vi "Keithley6221Monitor.vi"() -> ()   [LabVIEW 2019]
uses:
  Utility/Monitor Communication/K6221/K6221_Cluster.ctl
  Global/Global Variables/Data_Display_global.vi
  Instrument_Setup.vi
  Utility/Monitor Communication/sub-vis/K6221_Open_Queue.vi
  Utility/Monitor Communication/sub-vis/K6221_Check_Queue.vi
  <vilib>/ErrorRing/Error Ring.xnode
  Equipment/Keithley 622x/Keithley 622x.lvlib
panel:
  out "Cluster":T1
  # "K 6221"
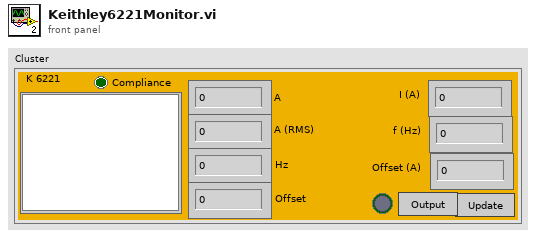
[diagram p1: front panel]
types:
  T1 = typedef "K6221_Cluster.ctl" = cluster{"Plot Window":dbl[][], "A":dbl, "A (RMS)":dbl, "Hz":dbl, "I (A)":dbl, "f (Hz)":dbl, "Update":bool, "Offset":dbl, "Offset (A)":dbl, "Compliance":bool, "Output":bool, "Output Status":bool}
  T2 = typedef "Keithley 622x.lvlib/KE622x -- Current Level.ctl" = dbl
  T3 = typedef "Keithley 622x.lvlib/KE622x -- On Off Control.ctl" = enum16{"Off", "On"}
  T4 = typedef "Keithley 622x.lvlib/KE6221 -- Wave Sine Wave Params.ctl" = cluster{"Frequency (Hz)":T5, "Amplitude (A)":T6, "Offset (A)":T2, "Ranging Mode":T7, "Fixed Range":T8, "Playback Mode":T9, "Time (s)":T10, "Num Cycles":T11, "Phase\nMarker?":bool, "Phase Marker (deg)":T12, "Trig Link Line":T13}
  T5 = typedef "Keithley 622x.lvlib/KE6221 -- Wave Frequency.ctl" = dbl
  T6 = typedef "Keithley 622x.lvlib/KE6221 -- Wave Amplitude.ctl" = dbl
  T7 = typedef "Keithley 622x.lvlib/KE6221 -- Wave Ranging Mode.ctl" = enum16{"Best", "Fixed"}
  T8 = typedef "Keithley 622x.lvlib/KE622x -- Current Ranges.ctl" = enum16{"2nA", "20nA", "200nA", "2uA", "20uA", "200uA", "2mA", "20mA", "100mA"}
  T9 = typedef "Keithley 622x.lvlib/KE6221 -- Wave Playback Mode.ctl" = enum16{"Time", "Num Cycles"}
  T10 = typedef "Keithley 622x.lvlib/KE6221 -- Wave Playback Time.ctl" = dbl
  T11 = typedef "Keithley 622x.lvlib/KE6221 -- Wave Playback Num Cycles.ctl" = dbl
  T12 = typedef "Keithley 622x.lvlib/KE6221 -- Wave Phase Marker.ctl" = dbl
  T13 = typedef "Keithley 622x.lvlib/KE622x -- Trig Link Line.ctl" = enum16{"1", "2", "3", "4", "5", "6"}
  T14 = typedef "Keithley 622x.lvlib/KE622x -- Current Range.ctl" = cluster{"Auto Range?":bool, "Man / Selected\nRange":T8}
  T15 = typedef "Keithley 622x.lvlib/KE622x -- Voltage Limit.ctl" = dbl
  T16 = typedef "Keithley 622x.lvlib/KE6221 -- Output Response.ctl" = enum16{"Fast", "Slow"}
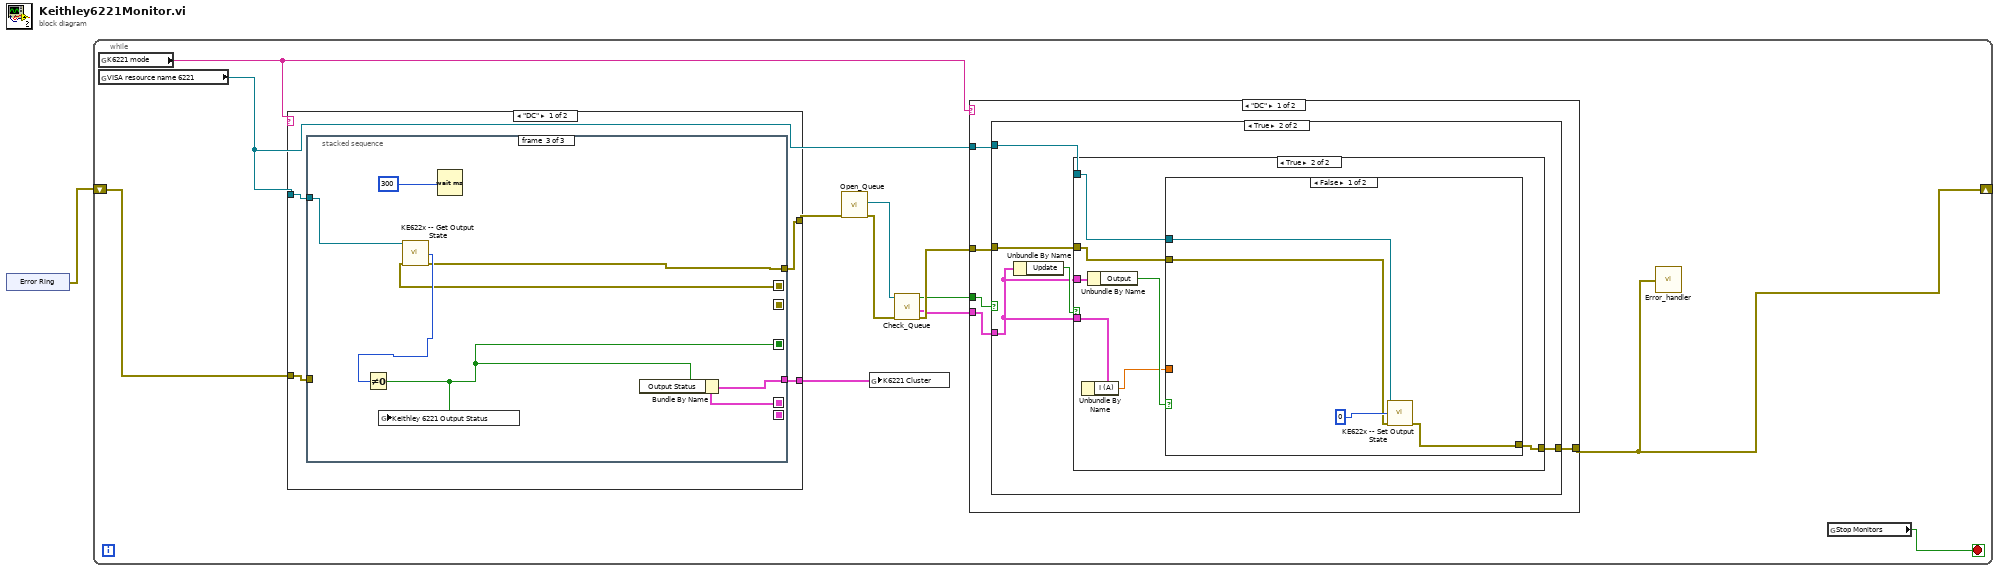
[diagram p0: block diagram]
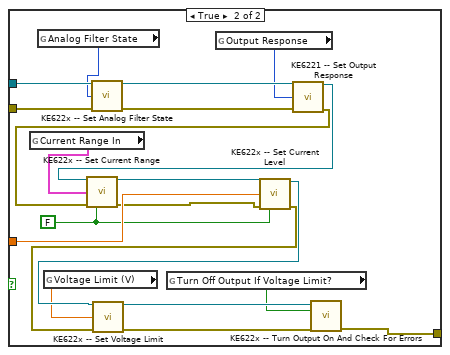
[diagram p4: hidden frame]
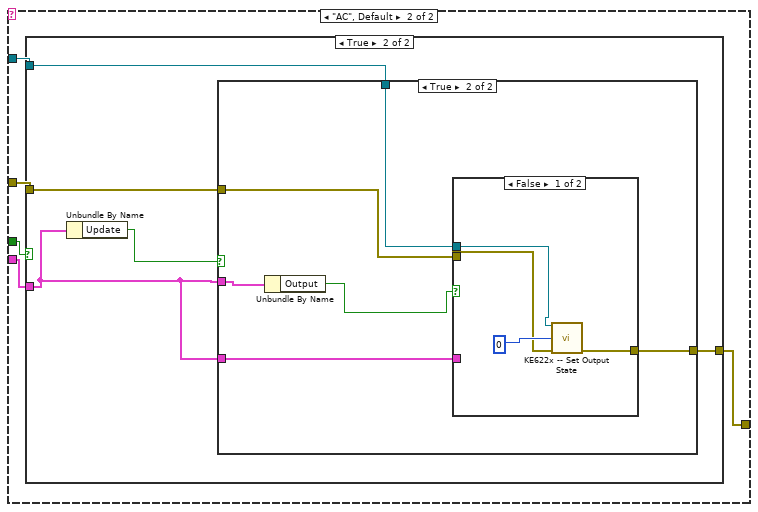
[diagram p5: hidden frame]
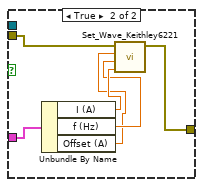
[diagram p8: hidden frame]
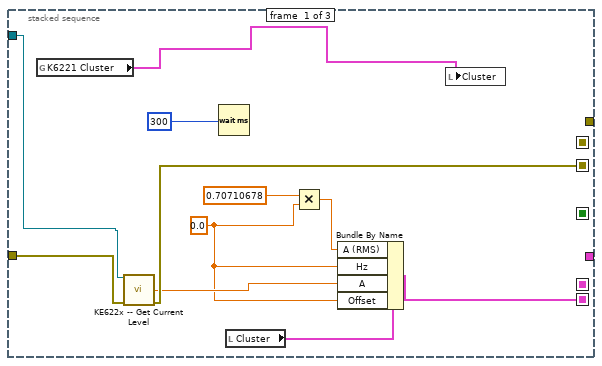
[diagram p9: hidden frame]
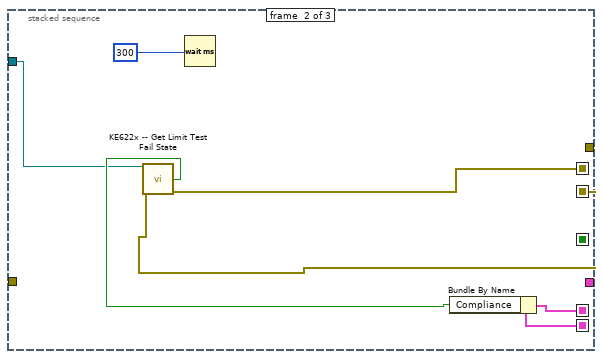
[diagram p10: hidden frame]
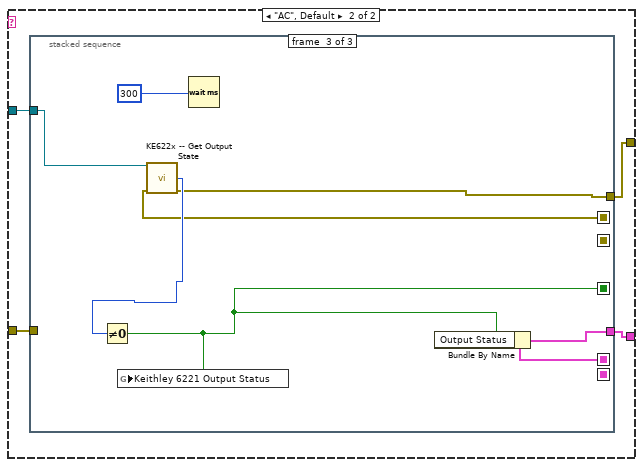
[diagram p11: hidden frame]
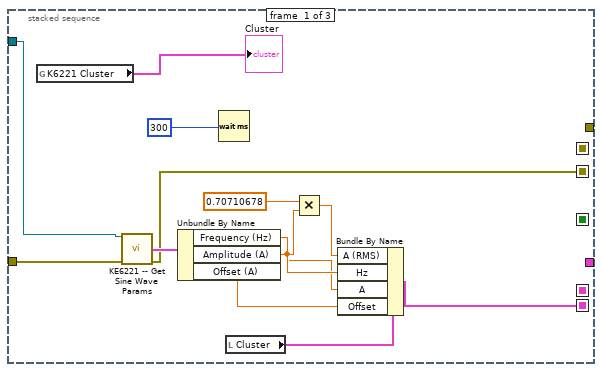
[diagram p12: hidden frame]
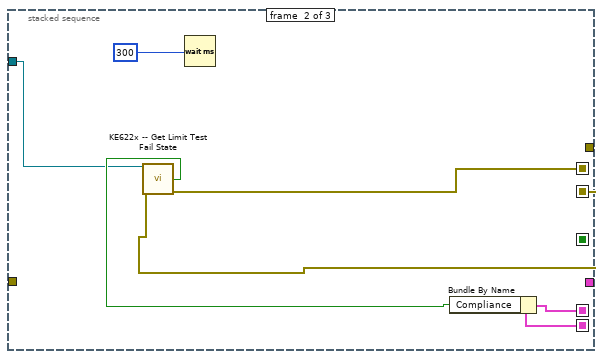
[diagram p13: hidden frame]
diagram:
  n1 = xnode "Error Ring"() -> ("error out"=w1:errorcluster)
  n2 = while {
    shift-right: [w4] -> _
    shift-left: w1 -> [w2]
    stop <- w13 stop-if-true
    n3 = global read "Instrument_Setup.vi" "K6221 mode"() -> (w3:string)
    n4 = global read "Instrument_Setup.vi" "VISA resource name 6221"() -> (w6:refnum<visa-resource-name>)
    n5 = case shown="\"DC\"" w3 {
      tunnel: w2 -> [w87 w118]
      tunnel: [w86 w117] -> w12
      tunnel: w6 -> [w88 w116]
      tunnel: [w85 w115] -> w5
      frame "DC" {
        n6 = stacked-sequence {
          seq-local: [w91 _ _] -> [_ w105 _]
          seq-local: [_ _ w111] -> [_ _ _]
          seq-local: [_ w100 _] -> [_ _ w109]
          seq-local: [w97 _ _] -> [_ w104 _]
          seq-local: [_ w103 _] -> [_ _ w112]
          tunnel: w88 -> [w93 w101 w110]
          tunnel: w87 -> [w92 _ _]
          tunnel: [_ _ w108] -> w86
          tunnel: [_ _ w107] -> w85
          frame #0 {
            w89 = 0.0
            n7 = global read "Data_Display_global.vi" "K6221 Cluster"() -> (w94:T1)
            n8 = call "KE622x -- Get Current Level.vi"("Resource In"=w93, "error in (no error)"=w92) -> ("Current Level (A)"=w90:T2, "error out"=w91:errorcluster)  [unwired: 11 in, 1 out]
            n9 = Wait (ms)(milliseconds to wait=300) -> ()  [unwired: 1 out]
            n10 = local read "Cluster"() -> (w98:T1)
            n11 = Multiply(x=0.70710678, y=w89) -> (x*y=w95:dbl)
            n12 = Bundle By Name(cluster=w98, "A (RMS)"=w95, "Hz"=w89, "A"=w90, "Offset"=w89) -> (w97:T1)
            n13 = local write "Cluster"(w94) -> ()
          }
          frame #1 {
            n14 = call "KE622x -- Get Limit Test Fail State.vi"("Resource In"=w101, "error in (no error)"=w105) -> ("Limit Test Failed (Compliance)?"=w102:bool, "error out"=w100:errorcluster)  [unwired: 11 in, 1 out]
            n15 = Wait (ms)(milliseconds to wait=300) -> ()  [unwired: 1 out]
            n16 = Bundle By Name(cluster=w104, "Compliance"=w102) -> (w103:T1)
          }
          frame #2 {
            n17 = call "KE622x -- Get Output State.vi"("Resource In"=w110, "error in (no error)"=w109) -> ("Output State"=w114:T3, "error out"=w108:errorcluster)  [unwired: 11 in, 1 out]
            n18 = Not Equal To 0?(x=w114) -> (x != 0?=w111:bool)
            n19 = global write "Data_Display_global.vi" "Keithley 6221 Output Status"(w111) -> ()
            n20 = Wait (ms)(milliseconds to wait=300) -> ()  [unwired: 1 out]
            n21 = Bundle By Name(cluster=w112, "Output Status"=w111) -> (w107:T1)
          }
        }
      }
      frame "AC", Default {
        n22 = stacked-sequence {
          seq-local: [w129 _ _] -> [_ w137 _]
          seq-local: [_ _ w143] -> [_ _ _]
          seq-local: [_ w132 _] -> [_ _ w141]
          seq-local: [w122 _ _] -> [_ w136 _]
          seq-local: [_ w135 _] -> [_ _ w144]
          tunnel: w116 -> [w125 w133 w142]
          tunnel: w118 -> [w124 _ _]
          tunnel: [_ _ w140] -> w117
          tunnel: [_ _ w139] -> w115
          frame #0 {
            n23 = global read "Data_Display_global.vi" "K6221 Cluster"() -> (→"Cluster":T1)
            n24 = call "KE6221 -- Get Sine Wave Params.vi"("Resource In"=w125, "error in (no error)"=w124) -> ("Sine Wave Params"=w131:T4, "error out"=w129:errorcluster)  [unwired: 11 in, 1 out]
            n25 = Unbundle By Name(w131) -> ("Frequency (Hz)"=w127:T5, "Amplitude (A)"=w121:T6, "Offset (A)"=w126:T2)
            n26 = Wait (ms)(milliseconds to wait=300) -> ()  [unwired: 1 out]
            n27 = local read "Cluster"() -> (w128:T1)
            n28 = Multiply(x=0.70710678, y=w121) -> (x*y=w119:T6)
            n29 = Bundle By Name(cluster=w128, "A (RMS)"=w119, "Hz"=w127, "A"=w121, "Offset"=w126) -> (w122:T1)
          }
          frame #1 {
            n30 = call "KE622x -- Get Limit Test Fail State.vi"("Resource In"=w133, "error in (no error)"=w137) -> ("Limit Test Failed (Compliance)?"=w134:bool, "error out"=w132:errorcluster)  [unwired: 11 in, 1 out]
            n31 = Wait (ms)(milliseconds to wait=300) -> ()  [unwired: 1 out]
            n32 = Bundle By Name(cluster=w136, "Compliance"=w134) -> (w135:T1)
          }
          frame #2 {
            n33 = call "KE622x -- Get Output State.vi"("Resource In"=w142, "error in (no error)"=w141) -> ("Output State"=w146:T3, "error out"=w140:errorcluster)  [unwired: 11 in, 1 out]
            n34 = Not Equal To 0?(x=w146) -> (x != 0?=w143:bool)
            n35 = global write "Data_Display_global.vi" "Keithley 6221 Output Status"(w143) -> ()
            n36 = Wait (ms)(milliseconds to wait=300) -> ()  [unwired: 1 out]
            n37 = Bundle By Name(cluster=w144, "Output Status"=w143) -> (w139:T1)
          }
        }
      }
    }
    n38 = call-poly "Open_Queue.vi"("error in (no error)"=w12) -> ("error out"=w11:errorcluster, "queue out"=w10:refnum<queue>)  [unwired: 9 in]
    n39 = global write "Data_Display_global.vi" "K6221 Cluster"(w5) -> ()
    n40 = call-poly "Check_Queue.vi"("error in (no error)"=w11, "queue"=w10) -> ("error out"=w9:errorcluster, "Command (in)"=w8:T1, "New Entries?"=w7:bool)  [unwired: 6 in]
    n41 = case shown="\"DC\"" w3 {
      tunnel: w9 -> [w16 w61]
      tunnel: w8 -> [w17 w60]
      tunnel: w7 -> [w18 w59]
      tunnel: w6 -> [w15 w58]
      tunnel: [w14 w57] -> w4
      frame "DC" {
        n42 = case shown="True" w18 {
          tunnel: w16 -> [w19 w22]
          tunnel: w17 -> [_ w21]
          tunnel: w15 -> [_ w23]
          tunnel: [w19 w20] -> w14
          frame False {
          }
          frame True {
            n43 = Unbundle By Name(w21) -> ("Update"=w24:bool)
            n44 = case shown="True" w24 {
              tunnel: w23 -> [_ w28]
              tunnel: w22 -> [w25 w26]
              tunnel: w21 -> [_ w32]
              tunnel: w21 -> [_ w31]
              tunnel: [w25 w29] -> w20
              frame False {
              }
              frame True {
                n45 = Unbundle By Name(w31) -> ("I (A)"=w27:dbl)
                n46 = Unbundle By Name(w32) -> ("Output"=w30:bool)
                n47 = case shown="False" w30 {
                  tunnel: [w35 w56] -> w29
                  tunnel: w28 -> [w33 w52]
                  tunnel: w27 -> [_ w46]
                  tunnel: w26 -> [w34 w45]
                  frame False {
                    n48 = call "KE622x -- Set Output State.vi"("Resource In"=w33, "Output State"=0, "error in (no error)"=w34) -> ("error out"=w35:errorcluster)  [unwired: 11 in, 1 out]
                  }
                  frame True {
                    w37 = FALSE ("Read Back Set Values? (T)")
                    n49 = global read "Instrument_Setup.vi" "Current Range In"() -> (w47:T14)
                    n50 = global read "Instrument_Setup.vi" "Analog Filter State"() -> (w49:T3)
                    n51 = global read "Instrument_Setup.vi" "Voltage Limit (V)"() -> (w38:T15)
                    n52 = call "KE622x -- Set Analog Filter State.vi"("Resource In"=w52, "Analog Filter State"=w49, "error in (no error)"=w45) -> ("Resource Out (dupl)"=w51:refnum<visa-resource-name>, "error out"=w44:errorcluster)  [unwired: 11 in]
                    n53 = global read "Instrument_Setup.vi" "Turn Off Output If Voltage Limit?"() -> (w53:bool)
                    n54 = global read "Instrument_Setup.vi" "Output Response"() -> (w48:T16)
                    n55 = call "KE6221 -- Set Output Response.vi"("Resource In"=w51, "KE6221 Output Response"=w48, "error in (no error)"=w44) -> ("Resource Out (dupl)"=w50:refnum<visa-resource-name>, "error out"=w43:errorcluster)  [unwired: 11 in]
                    n56 = call "KE622x -- Set Current Range.vi"("Resource In"=w50, "Current Range In"=w47, "error in (no error)"=w43, "Read Back Set Values? (T)"=w37) -> ("Resource Out (dupl)"=w40:refnum<visa-resource-name>, "error out"=w42:errorcluster)  [unwired: 9 in, 1 out]
                    n57 = call "KE622x -- Set Current Level.vi"("Resource In"=w40, "Current Level (A) In"=w46, "error in (no error)"=w42, "Read Back Set Value? (T)"=w37) -> ("Resource Out (dupl)"=w39:refnum<visa-resource-name>, "error out"=w41:errorcluster)  [unwired: 9 in, 1 out]
                    n58 = call "KE622x -- Set Voltage Limit.vi"("Resource In"=w39, "Voltage Limit (V)"=w38, "error in (no error)"=w41) -> ("Resource Out (dupl)"=w54:refnum<visa-resource-name>, "error out"=w55:errorcluster)  [unwired: 11 in]
                    n59 = call "KE622x -- Turn Output On And Check For Errors.vi"("Resource In"=w54, "Turn Off Output If Compliance?"=w53, "error in (no error)"=w55) -> ("error out"=w56:errorcluster)  [unwired: 9 in, 3 out]
                  }
                }
              }
            }
          }
        }
      }
      frame "AC", Default {
        n60 = case shown="True" w59 {
          tunnel: w61 -> [w62 w65]
          tunnel: w60 -> [_ w64]
          tunnel: w58 -> [_ w66]
          tunnel: [w62 w63] -> w57
          frame False {
          }
          frame True {
            n61 = Unbundle By Name(w64) -> ("Update"=w67:bool)
            n62 = case shown="True" w67 {
              tunnel: w66 -> [_ w74]
              tunnel: w65 -> [w68 w73]
              tunnel: w64 -> [_ w72]
              tunnel: w64 -> [_ w71]
              tunnel: [w68 w70] -> w63
              frame False {
              }
              frame True {
                n63 = Unbundle By Name(w72) -> ("Output"=w69:bool)
                n64 = case shown="False" w69 {
                  tunnel: w74 -> [w77 _]
                  tunnel: w73 -> [w76 w84]
                  tunnel: [w75 w83] -> w70
                  tunnel: w71 -> [_ w82]
                  frame False {
                    n65 = call "KE622x -- Set Output State.vi"("Resource In"=w77, "Output State"=0, "error in (no error)"=w76) -> ("error out"=w75:errorcluster)  [unwired: 11 in, 1 out]
                  }
                  frame True {
                    n66 = Unbundle By Name(w82) -> ("I (A)"=w81:dbl, "f (Hz)"=w80:dbl, "Offset (A)"=w79:dbl)
                    n67 = call "Set_Wave_Keithley6221.vi"("I (A)"=w81, "f (Hz)"=w80, "Offset (A)"=w79, "Error in"=w84) -> ("Erro out"=w83:errorcluster)  [unwired: 5 in]
                  }
                }
              }
            }
          }
        }
      }
    }
    n68 = call "Error_handler.vi"("error constant"=w4) -> ()
    n69 = global read "Data_Display_global.vi" "Stop Monitors"() -> (w13:bool)
  }
